vi "Select Active Channels.vi"(8 "error in (no error)":errorcluster, 10 "Active Channel(s)":T1[](array[typedef]), 11 "PicoScope 3000a in":refnum<class "PicoScope 3000a.lvclass">) -> (0 "error out":errorcluster, 3 "PicoScope 3000a out":refnum<class "PicoScope 3000a.lvclass">)   [LabVIEW 2018, in "PicoScope 3000a.lvlib" / "PicoScope 3000a.lvclass"]
doc: "This Override method is used to set active channels for the Oscope. Use the 'Active Channel(s)' control to select channel(s)."
uses:
  PicoScope 3000a.lvclass
  PPLs/Oscilloscope/Parent/Oscilloscope.lvlibp/Custom Controls/Analog Channels.ctl
  PicoScope 3000a.lvclass/PicoScope 3000a.ctl
  PPLs/Oscilloscope/Parent/Oscilloscope.lvlibp
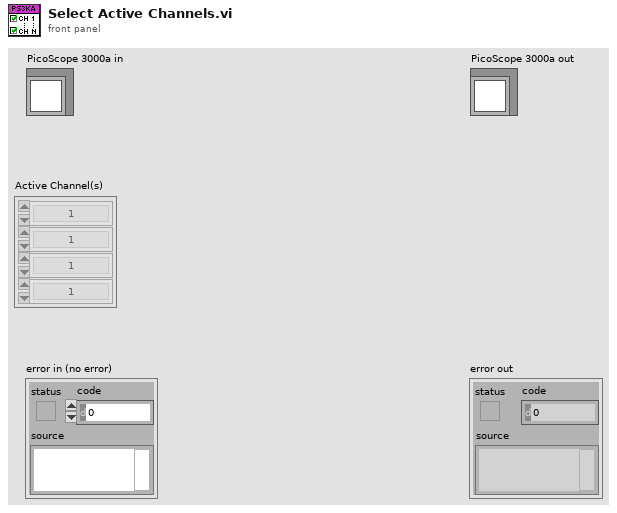
[diagram p1: front panel]
types:
  T1 = typedef "Oscilloscope.lvlibp/Analog Channels.ctl" = enum16{"1", "2", "3", "4", "5", "6", "7", "8", "9", "10", "11", "12", "13", "14", "15", "16"}
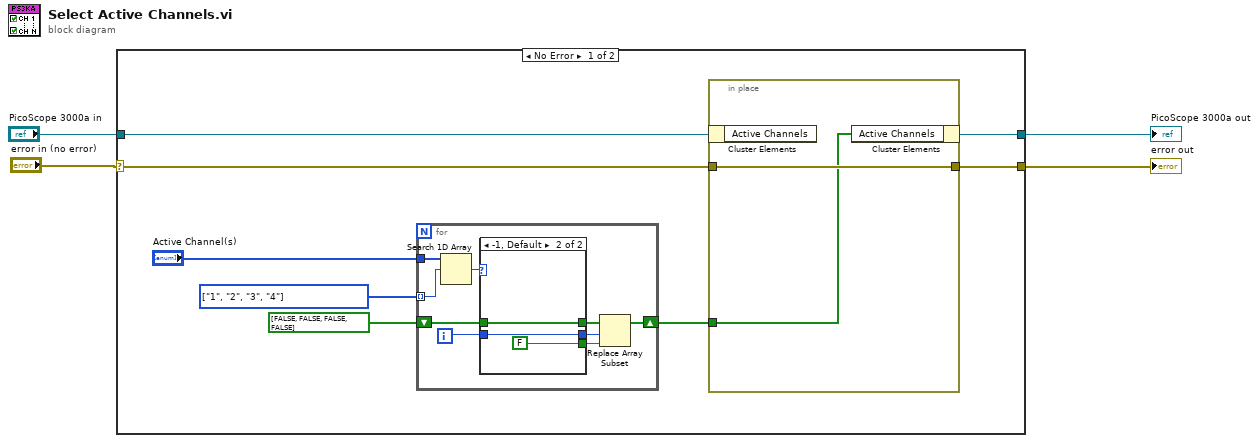
[diagram p0: block diagram]
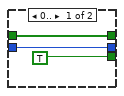
[diagram p2: hidden frame]
diagram:
  n1 = case shown="No Error" "error in (no error)" {
    selector: "error in (no error)" -> [w8 w30]
    tunnel: "PicoScope 3000a in" -> [w7 w31]
    tunnel: [w6 w31] -> w2
    tunnel: [w5 w30] -> w1
    frame No Error {
      w10 = T1[] [enum."1", enum."2", enum."3", enum."4"] items=["1", "2", "3", "4", "5", "6", "7", "8", "9", "10", "11", "12", "13", "14", "15", "16"] ("Active Channel(s)")
      n2 = for {
        tunnel: "Active Channel(s)" -> [w22]
        shift-right: [w18] -> w9
        shift-left: bool[] [FALSE, FALSE, FALSE, FALSE] -> [w20]
        tunnel: w10 -> [w23] mode=indexing
        i -> [w15]
        n3 = Search 1D Array(1D array=w22, element=w23) -> (index of element=w21:i32)  [unwired: 1 in]
        n4 = case shown="-1, Default" w21 {
          tunnel: w20 -> [w26 w29]
          tunnel: [w26 w29] -> w19
          tunnel: [TRUE ("new element/subarray") FALSE ("new element/subarray")] -> w17
          tunnel: [w24 w27] -> w16
          tunnel: w15 -> [w24 w27]
          frame 0.. {
          }
          frame -1, Default {
          }
        }
        n5 = Replace Array Subset(array=w19, new element=w17, index=w16) -> (w18:bool[])
      }
      n6 = in-place {
        in-place-border: w8 -> [w14]
        in-place-border: [w14] -> w5
        in-place-border: w9 -> [w13]
        n7 = in-place-cluster #1(w7) -> ()  [unwired: 1 out]
        n8 = in-place-cluster #1("Active Channels"=w13) -> (w6:refnum<class "PicoScope 3000a.lvclass">)
      }
    }
    frame Error {
    }
  }
  "error out" <- w1
  "PicoScope 3000a out" <- w2
